vi "Create GCentral External URL Pages.vi"() -> ()   [LabVIEW 2020]
uses:
  Libraries/Packages/Repo_class/Repo.lvclass/Repo.ctl
  Libraries/Packages/Package_class/Package.lvclass/Package.ctl
  Libraries/Packages/Package Version_class/Package Version.lvclass/Package Version.ctl
  Libraries/Packages/Package_class/Read DisplayName.vi
  Libraries/Packages/Package_class/Read Name.vi
  Libraries/Packages/Package_class/Read Versions.vi
  Libraries/Packages/Package Version_class/Read Name.vi
  Libraries/Packages/Package Version_class/Read ReleaseDate.vi
  Libraries/Packages/Package Version_class/Read Summary.vi
  Libraries/Packages/Package Version_class/Read Description.vi
  Libraries/Packages/Package Version_class/Read Vendor.vi
  Libraries/Packages/Package Version_class/Read Author.vi
  Libraries/Packages/Package Version_class/Read IconURL.vi
  Libraries/Packages/Repo_class/Read Packages.vi
  Libraries/Packages/Package_class/Package.lvclass
  Libraries/Packages/Package Version_class/Package Version.lvclass
  Libraries/WSsupport/WSsupport.lvlib
  Libraries/Packages/Repo_class/Repo.lvclass
panel:
  out "Downloaded Image":picture
  out "File Markdown Text":string
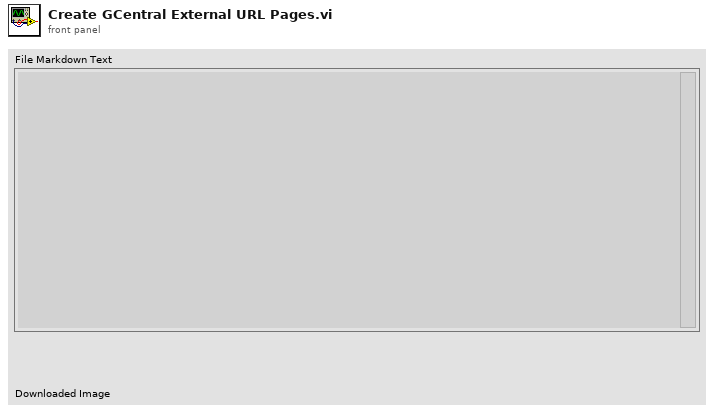
[diagram p1: front panel]
types:
  T1 = typedef "imagedata.ctl" = cluster{"image type":i32, "image depth":i32, "image":u8[], "mask":u8[], "colors":u32[], "Rectangle":cluster{"left":i16, "top":i16, "right":i16, "bottom":i16}}
  T2 = cluster{"left":i16, "top":i16, "right":i16, "bottom":i16}
  T3 = cluster{"Horizontal Shift":i16, "Vertical Shift":i16}
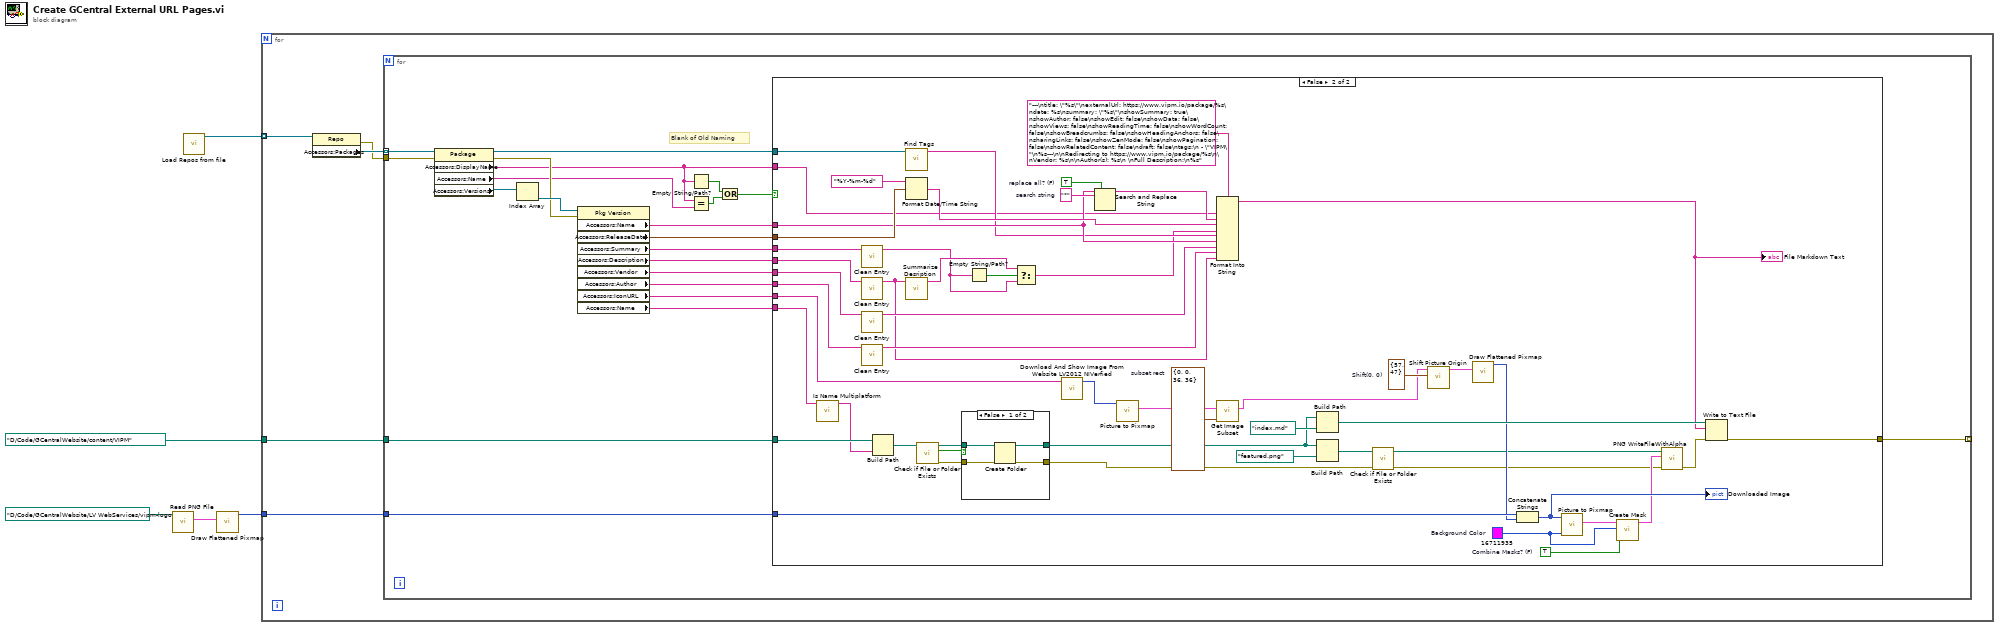
[diagram p0: block diagram]
diagram:
  n1 = call <vilib>:"Read PNG File.vi"("path to PNG file"=path "D:/Code/GCentralWebsite/LV WebServices/vipm-logo.png") -> ("image data"=w2:T1)  [unwired: 8 in, 2 out]
  n2 = call "Load Repos from file.vi"() -> ("Repos"=w5:refnum<class "Repo.lvclass">[])  [unwired: 10 in, 1 out]
  n3 = call <vilib>:"Draw Flattened Pixmap.vi"("image data"=w2) -> ("new picture"=w1:picture)  [unwired: 8 in]
  n4 = for {
    tunnel: w5 -> [w10] mode=indexing
    tunnel: path "D:/Code/GCentralWebsite/content/VIPM" -> [w8]
    tunnel: w1 -> [w7]
    n5 = property class="Repo"(reference=w10) -> (error out=w6:errorcluster, "Accessors:Packages"=w9:refnum<class "Package.lvclass">[])  [unwired: 1 in, 1 out]
    n6 = for {
      tunnel: w9 -> [w21] mode=indexing
      tunnel: w8 -> [w28]
      tunnel: [w32] -> _ mode=indexing
      tunnel: w7 -> [w19]
      tunnel: w6 -> [w18]
      # "Blank of Old Naming"
      n7 = property class="Package"(reference=w21, error in=w18) -> (reference out=w20:refnum<class "Package.lvclass">, error out=w17:errorcluster, "Accessors:DisplayName"=w15:string, "Accessors:Name"=w16:string, "Accessors:Versions"=w31:refnum<class "Package Version.lvclass">[])
      n8 = Index Array(array=w31) -> (element=w30:refnum<class "Package Version.lvclass">)  [unwired: 1 in]
      n9 = property class="Pkg Version"(reference=w30, error in=w17) -> ("Accessors:Name"=w22:string, "Accessors:ReleaseDate"=w23:timestamp, "Accessors:Summary"=w11:string, "Accessors:Description"=w26:string, "Accessors:Vendor"=w25:string, "Accessors:Author"=w24:string, "Accessors:IconURL"=w27:string, "Accessors:Name"=w29:string)  [unwired: 2 out]
      n10 = Empty String/Path?(string/path=w15) -> (empty?=w14:bool)
      n11 = Equal?(x=w15, y=w16) -> (x = y?=w13:bool)
      n12 = Or(x=w14, y=w13) -> (x .or. y?=w12:bool)
      n13 = case shown="False" w12 {
        tunnel: [_ w85] -> w32
        tunnel: w29 -> [_ w82]
        tunnel: w28 -> [_ w81]
        tunnel: w27 -> [_ w76]
        tunnel: w26 -> [_ w60]
        tunnel: w25 -> [_ w57]
        tunnel: w24 -> [_ w56]
        tunnel: w23 -> [_ w63]
        tunnel: w22 -> [_ w59]
        tunnel: w20 -> [_ w54]
        tunnel: w19 -> [_ w51]
        tunnel: w15 -> [_ w41]
        tunnel: w11 -> [_ w34]
        frame True {
        }
        frame False {
          w38 = T2 {"left"=0, "top"=0, "right"=36, "bottom"=36}  # subset rect
          w46 = TRUE  # Combine Masks? (F)
          w47 = u32 16711935  # Background Color
          w53 = T3 {"Horizontal Shift"=57, "Vertical Shift"=47}  # Shift(0, 0)
          w68 = TRUE  # replace all? (F)
          w69 = "*"  # search string
          n14 = call <vilib>:"Is Name Multiplatform.vi"("filename"=w82) -> ("suggested filename"=w80:string)  [unwired: 6 in, 4 out]
          n15 = call "Clean Entry.vi"("string in"=w34) -> ("string out"=w33:string)  [unwired: 10 in]
          n16 = call "Clean Entry.vi"("string in"=w60) -> ("string out"=w58:string)  [unwired: 10 in]
          n17 = call "Clean Entry.vi"("string in"=w57) -> ("string out"=w66:string)  [unwired: 10 in]
          n18 = call "Clean Entry.vi"("string in"=w56) -> ("string out"=w65:string)  [unwired: 10 in]
          n19 = Build Path(base path=w81, name or relative path=w80) -> (appended path=w79:path)
          n20 = call "Find Tags.vi"("Package"=w54) -> ("Tags Front Matter"=w55:string)  [unwired: 10 in]
          n21 = Format Date/Time String(time format string (%c)="%Y-%m-%d", seconds (now)=w63) -> (date/time string=w61:string)  [unwired: 1 in]
          n22 = call "Summarize Desription.vi"("Description in"=w58) -> ("Summary out"=w36:string)  [unwired: 10 in]
          n23 = call <vilib>:"Check if File or Folder Exists.vi"("path"=w79) -> ("error out"=w86:errorcluster, "file or folder exists?"=w78:bool, "dup path"=w77:path)  [unwired: 8 in]
          n24 = case shown="False" w78 {
            tunnel: w77 -> [w88 w91]
            tunnel: [w87 w91] -> w70
            tunnel: w86 -> [w90 w92]
            tunnel: [w89 w92] -> w84
            frame False {
              n25 = Create Folder(path (use dialog)=w88, error in=w90) -> (created path=w87:path, error out=w89:errorcluster)  [unwired: 1 in, 1 out]
            }
            frame True {
            }
          }
          n26 = Empty String/Path?(string/path=w33) -> (empty?=w37:bool)
          n27 = Select(t=w36, s=w37, f=w33) -> (s? t:f=w35:string)
          n28 = call "Download And Show Image From Website LV2012 NIVerfied.vi"("Image URL"=w76) -> ("Downloaded Image"=w75:picture)  [unwired: 10 in]
          n29 = Search and Replace String(replace all?=w68, input string=w59, search string=w69) -> (result string=w67:string)  [unwired: 5 in, 3 out]
          n30 = call <vilib>:"Picture to Pixmap.vi"("picture"=w75) -> ("image data"=w40:T1)  [unwired: 9 in, 1 out]
          n31 = Format Into String(format string="---\ntitle: \"%s\"\nexternalUrl: https://www.vipm.io/package/%s\ndate: %s\nsummary: \"%s\"\nshowSummary: true\nshowAuthor: false\nshowEdit: false\nshowData: false\nshowViews: false\nshowReadingTime: false\nshowWordCount: false\nshowBreadcrumbs: false\nshowHeadingAnchors: false\nsharingLinks: false\nshowZenMode: false\nshowPagination: false\nshowRelatedContent: false\ndraft: false\ntags:\n - \"VIPM\"\n%s---\n\nRedirecting to https://www.vipm.io/package/%s\n\nVendor: %s\n\nAuthor(s): %s\n \nFull Description:\n%s", w41, w67, w61, w35, w55, w59, w66, w65, w58) -> (resulting string=w71:string)  [unwired: 2 in, 1 out]
          "File Markdown Text" <- w71
          n32 = call <vilib>:"Get Image Subset.vi"("subset rect"=w38, "image data"=w40) -> ("image subset"=w39:T1)  [unwired: 4 in, 1 out]
          n33 = Build Path(base path=w70, name or relative path=path "index.md") -> (appended path=w72:path)
          n34 = Build Path(base path=w70, name or relative path=path "featured.png") -> (appended path=w64:path)
          n35 = call <vilib>:"Check if File or Folder Exists.vi"("error in (no error)"=w84, "path"=w64) -> ("error out"=w43:errorcluster, "dup path"=w45:path)  [unwired: 7 in, 1 out]
          n36 = call "Shift Picture Origin.vi"("Shift(0, 0)"=w53, "image data IN"=w39) -> ("image data OUT"=w52:T1)  [unwired: 8 in, 1 out]
          n37 = call <vilib>:"Draw Flattened Pixmap.vi"("image data"=w52) -> ("new picture"=w50:picture)  [unwired: 8 in]
          n38 = Concatenate Strings(w51, w50) -> (w49:picture)
          "Downloaded Image" <- w49
          n39 = call <vilib>:"Picture to Pixmap.vi"("Background Color"=w47, "picture"=w49) -> ("image data"=w48:T1)  [unwired: 8 in, 1 out]
          n40 = call <vilib>:"Create Mask.vi"("Combine Masks? (F)"=w46, "Mask Color (Black)"=w47, "image data"=w48) -> ("image data"=w44:T1)  [unwired: 8 in]
          n41 = call "PNG WriteFileWithAlpha.vi"("error in (no error)"=w43, "image data"=w44, "Path to write (dialog)"=w45) -> ("error out"=w42:errorcluster)  [unwired: 7 in, 1 out]
          n42 = Write to Text File(file (use dialog)=w72, text=w71, error in=w42) -> (error out=w85:errorcluster)  [unwired: 1 in, 2 out]
        }
      }
    }
  }
